vi "rad_Modify AppImage Files.vi"(4 "Bitfiles Modified?":bool, 5 "Temp Image Folder":path, 6 "New Image?":bool, 7 "App Image Info File Path":path, 8 "error in (no error)":errorcluster, 10 "FPGA Properties":T1, 11 "AppImage Path":path) -> (0 "error out":errorcluster, 3 "AppImage Path Out":path)   [LabVIEW 2020]
uses:
  TypeDefs/rad_FPGA Properties.ctl
  TypeDefs/rad_FPGA Flash Properties.ctl
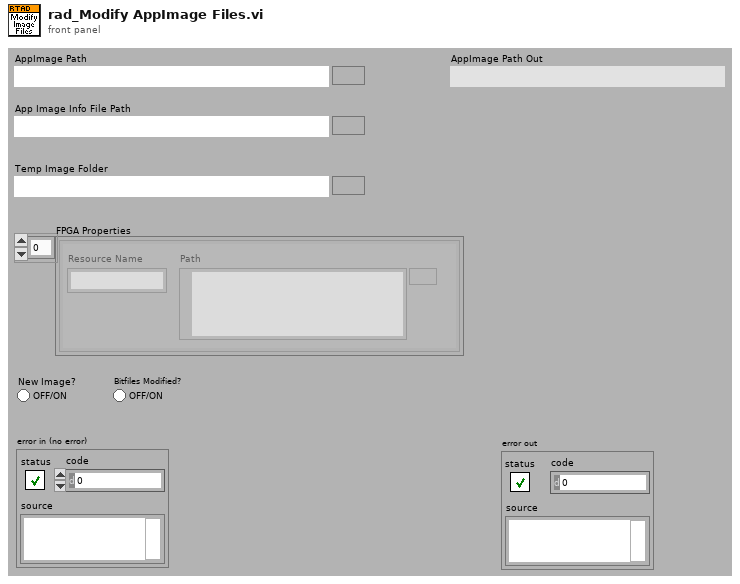
[diagram p1: front panel]
types:
  T1 = typedef "rad_FPGA Properties.ctl" = T2[]
  T2 = typedef "rad_FPGA Flash Properties.ctl" = cluster{"Resource Name":string, "Path":path}
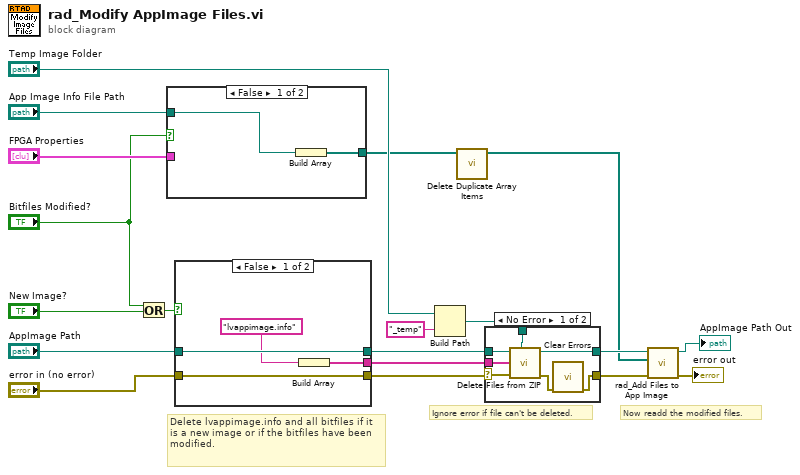
[diagram p0: block diagram]
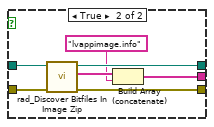
[diagram p3: hidden frame]
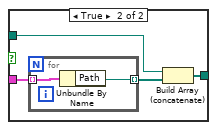
[diagram p4: hidden frame]
diagram:
  # "Ignore error if file can't be deleted."
  # "Now readd the modified files."
  # "Delete lvappimage.info and all bitfiles if it is a new image or if the bitfiles have been modified."
  n1 = Or(x="Bitfiles Modified?", y="New Image?") -> (x .or. y?=w3:bool)
  n2 = case shown="False" "Bitfiles Modified?" {
    tunnel: [w20 w25] -> w11
    tunnel: "App Image Info File Path" -> [w21 w24]
    tunnel: "FPGA Properties" -> [_ w23]
    frame False {
      n3 = Build Array(w21) -> (w20:path[])
    }
    frame True {
      n4 = for {
        tunnel: [w27] -> w22 mode=indexing
        tunnel: w23 -> [w26] mode=indexing
        n5 = Unbundle By Name(w26) -> ("Path"=w27:path)
      }
      n6 = Build Array (concatenate)(w24, w22) -> (w25:path[])
    }
  }
  n7 = case shown="False" w3 {
    tunnel: [w28 w32] -> w6
    tunnel: [w31 w38] -> w2
    tunnel: [w30 w37] -> w9
    tunnel: "AppImage Path" -> [w30 w36]
    tunnel: "error in (no error)" -> [w31 w35]
    frame False {
      n8 = Build Array("lvappimage.info" ("name or relative path")) -> (w28:string[])
    }
    frame True {
      n9 = call "rad_Discover Bitfiles In Image Zip.vi"("error in (no error)"=w35, "Image Path"=w36) -> ("error out"=w38:errorcluster, "Bitfiles Found"=w34:string[], "Image Path Out"=w37:path)  [unwired: 7 in]
      n10 = Build Array (concatenate)(w34, "lvappimage.info" ("name or relative path")) -> (w32:string[])
    }
  }
  n11 = Build Path(base path="Temp Image Folder", name or relative path="_temp") -> (appended path=w7:path)
  n12 = call "Delete Duplicate Array Items.vi"("Files"=w11) -> ("Files"=w10:path[])  [unwired: 10 in]
  n13 = case shown="No Error" w2 {
    selector: w2 -> [w41 w47]
    tunnel: [w45 w46] -> w19
    tunnel: w9 -> [w44 w46]
    tunnel: w7 -> [w43 _]
    tunnel: w6 -> [w42 _]
    tunnel: [w39 w47] -> w1
    frame No Error {
      n14 = call "Delete Files from ZIP.vi"("Temp Folder"=w43, "error in"=w41, "Files to Remove"=w42, "Zip File Path"=w44) -> ("error out"=w40:errorcluster, "Zip File Path Out"=w45:path)  [unwired: 6 in]
      n15 = call <vilib>:"Clear Errors.vi"("error in (no error)"=w40) -> ("error out"=w39:errorcluster)  [unwired: 5 in, 1 out]
    }
    frame Error {
    }
  }
  n16 = call "rad_Add Files to App Image.vi"("error in (no error)"=w1, "Files to Add"=w10, "AppImage Path"=w19) -> ("error out"=→"error out":errorcluster, "AppImage Path"=→"AppImage Path Out":path)  [unwired: 4 in, 3 out]
